vi "String Tuning low E.vi"(8 "Upper Limit":dbl, 9 "Lower Limit":dbl, 11 "Input Cluster":T1={"Tuner"={"Sharp"=FALSE, "Sharp"=FALSE, "Tuned"=FALSE, "Flat"=FALSE, "Flat"=FALSE}, "Chord"={"A"=FALSE, "B"=FALSE, "C"=FALSE, "D"=FALSE, "E"=FALSE, "F 2"=FALSE, "G"=FALSE}, "Note"={"Low E"=FALSE, "A"=FALSE, "D"=FALSE, "G"=FALSE, "B"=FALSE, "High E"=FALSE}, "Frequency Spectrum 2"=[{"t0"=timestamp(3721854148.349081 s since 1904-01-01), "dt"=0.0003333, "Y"=array[1000 elements], "attributes"=variant("NI_ChannelName"=variant(string "Voltage"), "NI_UnitDescription"=variant(string "Volts"))}]}) -> (1 "Tuned":bool, 3 "Output Cluster":T1={"Tuner"={"Sharp"=FALSE, "Sharp"=FALSE, "Tuned"=FALSE, "Flat"=FALSE, "Flat"=FALSE}, "Chord"={"A"=FALSE, "B"=FALSE, "C"=FALSE, "D"=FALSE, "E"=FALSE, "F 2"=FALSE, "G"=FALSE}, "Note"={"Low E"=FALSE, "A"=FALSE, "D"=FALSE, "G"=FALSE, "B"=FALSE, "High E"=FALSE}, "Frequency Spectrum 2"=[{"t0"=timestamp(3721854148.349081 s since 1904-01-01), "dt"=0.0003333, "Y"=array[1000 elements], "attributes"=variant("NI_ChannelName"=variant(string "Voltage"), "NI_UnitDescription"=variant(string "Volts"))}]})   [LabVIEW 2020]
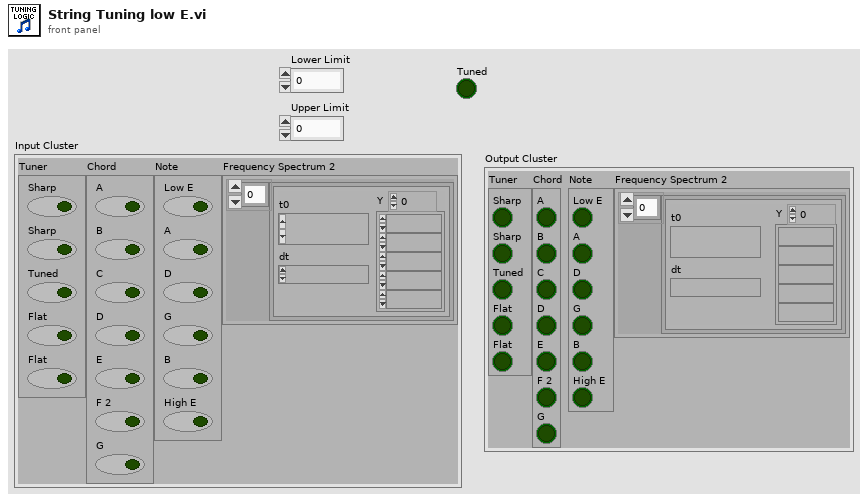
[diagram p1: front panel]
types:
  T1 = cluster{"Tuner":cluster{"Sharp":bool, "Sharp":bool, "Tuned":bool, "Flat":bool, "Flat":bool}, "Chord":cluster{"A":bool, "B":bool, "C":bool, "D":bool, "E":bool, "F 2":bool, "G":bool}, "Note":cluster{"Low E":bool, "A":bool, "D":bool, "G":bool, "B":bool, "High E":bool}, "Frequency Spectrum 2":dynamicdata}
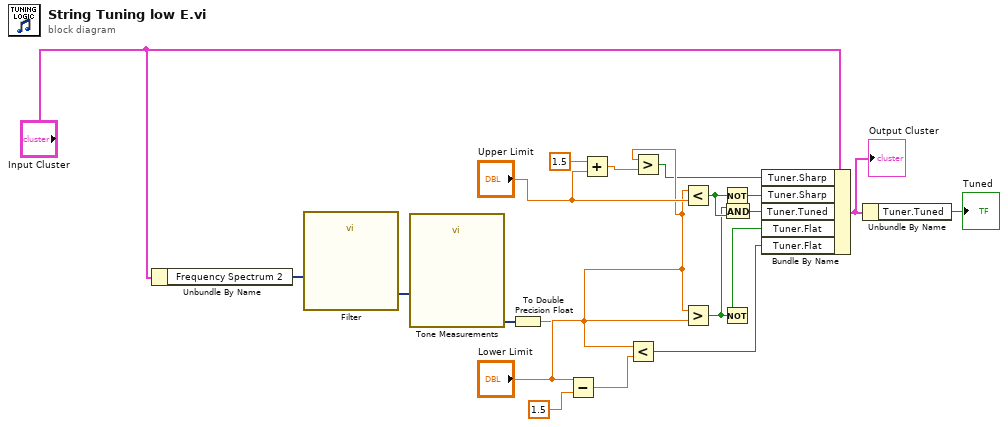
[diagram p0: block diagram]
diagram:
  n1 = Unbundle By Name("Input Cluster") -> ("Frequency Spectrum 2"=w13:dynamicdata)
  n2 = call "Filter"("Signal"=w13) -> ("Filtered Signal"=w14:dynamicdata)  [unwired: 9 in, 1 out]
  n3 = call "Tone Measurements"("Signals"=w14) -> ("Frequency"=w12:dynamicdata)  [unwired: 9 in, 1 out]
  n4 = To Double Precision Float(number=w12) -> (double precision float=w2:dbl)
  n5 = Subtract(x="Lower Limit", y=1.5) -> (x-y=w6:dbl)
  n6 = Add(x=1.5, y="Upper Limit") -> (x+y=w3:dbl)
  n7 = Less?(x=w2, y=w6) -> (x < y?=w7:bool)
  n8 = Greater?(x=w2, y=w3) -> (0:w1:bool)
  n9 = Less?(x=w2, y="Upper Limit") -> (x < y?=w19:bool)
  n10 = Greater?(x=w2, y="Lower Limit") -> (0:w17:bool)
  n11 = Not(x=w19) -> (.not. x?=w20:bool)
  n12 = Not(x=w17) -> (.not. x?=w18:bool)
  n13 = And(x=w17, y=w19) -> (x .and. y?=w16:bool)
  n14 = Bundle By Name(cluster="Input Cluster", "Tuner.Sharp"=w1, "Tuner.Sharp"=w20, "Tuner.Tuned"=w16, "Tuner.Flat"=w18, "Tuner.Flat"=w7) -> (w10:T1)
  "Output Cluster" <- w10
  n15 = Unbundle By Name(w10) -> ("Tuner.Tuned"=→"Tuned":bool)
